vi "Calculate Circle.vi"(7 "Display":bool, 9 "steps":i32=36, 10 "Circle":T1 {"Radius" format="%.2f"; "Center"."Y" format="%.2f"; "Center"."X" format="%.2f"}) -> (1 "Diameter":dbl, 2 "Circle Coordinates":cluster{"X":i32, "Y":i32}[](array[cluster]), 4 "y position":dbl, 6 "x position":dbl)   [LabVIEW 2013]
panel:
  out "r":dbl
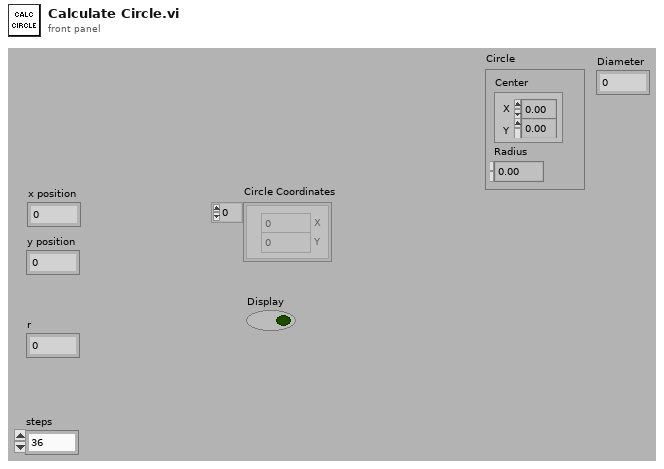
[diagram p1: front panel]
types:
  T1 = cluster{"Center":cluster{"X":sgl, "Y":sgl}, "Radius":dbl}
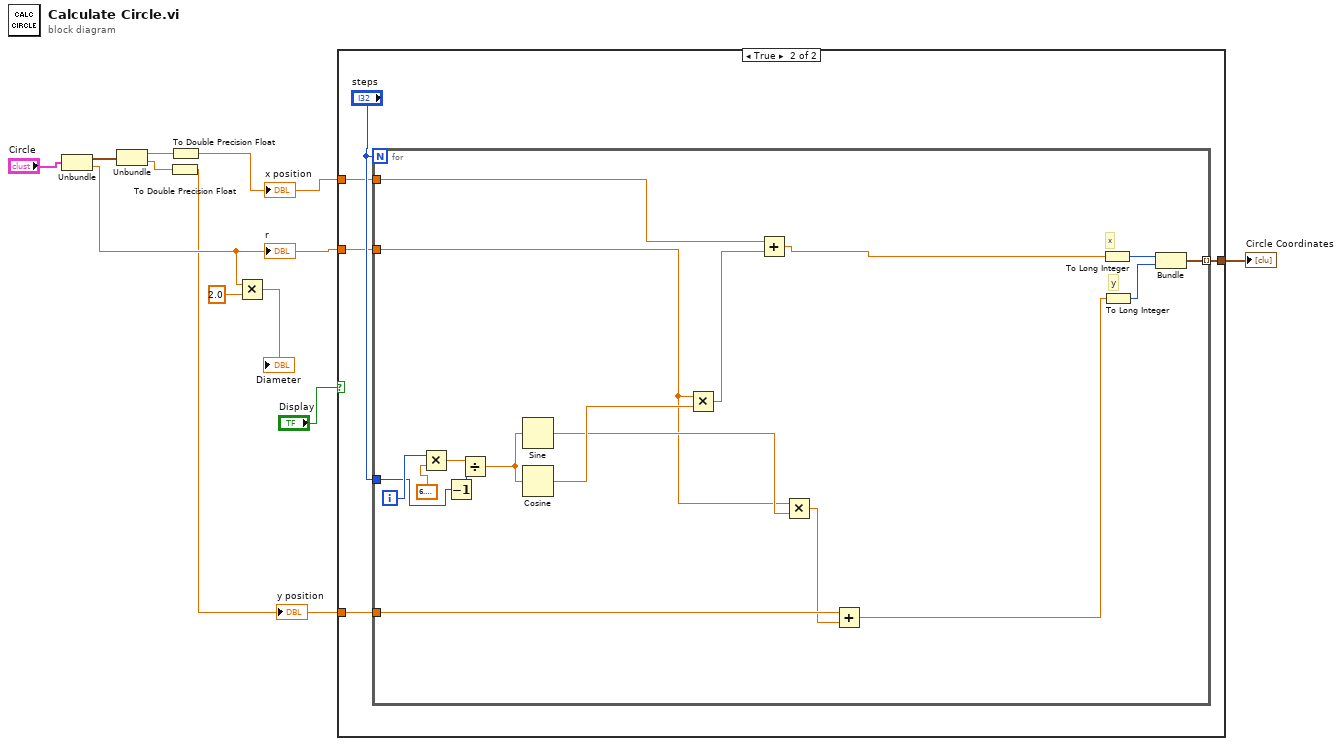
[diagram p0: block diagram]
diagram:
  n1 = Unbundle("Circle") -> ("Center"=w9:cluster{"X":sgl, "Y":sgl}, "Radius"=w8:dbl)
  "r" <- w8
  n2 = Unbundle(w9) -> ("X"=w5:sgl, "Y"=w4:sgl)
  n3 = To Double Precision Float(number=w4) -> (double precision float=w3:dbl)
  "y position" <- w3
  n4 = To Double Precision Float(number=w5) -> (double precision float=w2:dbl)
  "x position" <- w2
  n5 = Multiply(x=w8, y=2.0) -> (x*y=→"Diameter":dbl)
  n6 = case shown="True" "Display" {
    tunnel: [_ w16] -> w11
    tunnel: w8 -> [_ w14]
    tunnel: w3 -> [_ w13]
    tunnel: w2 -> [_ w12]
    frame False {
    }
    frame True {
      n7 = for {
        N: "steps" -> [_]
        tunnel: [w34] -> w16 mode=indexing
        tunnel: "steps" -> [w20]
        tunnel: w12 -> [w29]
        tunnel: w13 -> [w25]
        tunnel: w14 -> [w17]
        i -> [w33]
        # "y"
        # "x"
        n8 = Multiply(x=w33, y=6.283185307179586) -> (x*y=w32:dbl)
        n9 = Decrement(x=w20) -> (x-1=w19:i32)
        n10 = Divide(x=w32, y=w19) -> (x/y=w30:dbl)
        n11 = Sine(x=w30) -> (sin(x)=w22:dbl)
        n12 = Cosine(x=w30) -> (cos(x)=w26:dbl)
        n13 = Multiply(x=w17, y=w26) -> (x*y=w28:dbl)
        n14 = Add(x=w29, y=w28) -> (x+y=w18:dbl)
        n15 = Multiply(x=w17, y=w22) -> (x*y=w21:dbl)
        n16 = Add(x=w25, y=w21) -> (x+y=w24:dbl)
        n17 = To Long Integer(number=w18) -> (32bit integer=w27:i32)
        n18 = To Long Integer(number=w24) -> (32bit integer=w23:i32)
        n19 = Bundle(w27, w23) -> (w34:cluster{i32, i32})  [unwired: 1 in]
      }
    }
  }
  "Circle Coordinates" <- w11
